vi "Ultimus.vi"   [LabVIEW 2016, in "Assembly Tray.lvclass"]
uses:
  Classes/Workspace/Carrier Tray/Assembly Tray.lvclass
  Classes/Controller/Dispenser/Ultimus V/Ultimus V.lvclass
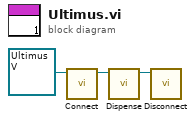
[diagram p0: block diagram]
diagram:
  n1 = call-dynamic "Connect.vi"("Ultimus V in"=refnum<class "Ultimus V.lvclass"> refnum ("Ultimus V.lvclass")) -> ("Ultimus V out"=w2:refnum<class "Ultimus V.lvclass">)  [unwired: 9 in, 1 out]
  n2 = call-dynamic "Dispense.vi"("Ultimus V in"=w2) -> ("Ultimus V out"=w1:refnum<class "Ultimus V.lvclass">)  [unwired: 9 in, 1 out]
  n3 = call-dynamic "Disconnect.vi"("Ultimus V in"=w1) -> ()  [unwired: 9 in, 1 out]
